vi "SID_1804453_labview_simulation.vi"() -> ()   [LabVIEW 2019]
uses:
  <vilib>/measure/matone.llb/Extract Single Tone Information N Chan.vi
  <vilib>/express/express analysis/Spectral/Block/exnSpectralBlock spectral measurements peak poly.vi
  <vilib>/express/express analysis/Spectral/Block/exnSpectralBlock spectral measurements peak DDT.vi
  <vilib>/express/express analysis/Spectral/XNode/ExpressSpectralMeasurementsBlockNode.xnode
  <vilib>/measure/NI_MAPro.lvlib
panel:
  out "Summing output graph":dynamicdata(graph)
  in  "Frequency":dbl=100.0
  in  "Amplitude":dbl=10.0
  out "peak output":dynamicdata(graph)
  in  "Time Target (s)":dbl=100.0
  out "Elapsed Time (s)":dbl
  in  "Ideal amplitude":dbl
  out "Out of bounds - amplitude":bool
  in  "Ideal frequency":dbl
  out "Out of bounds - frequency":bool
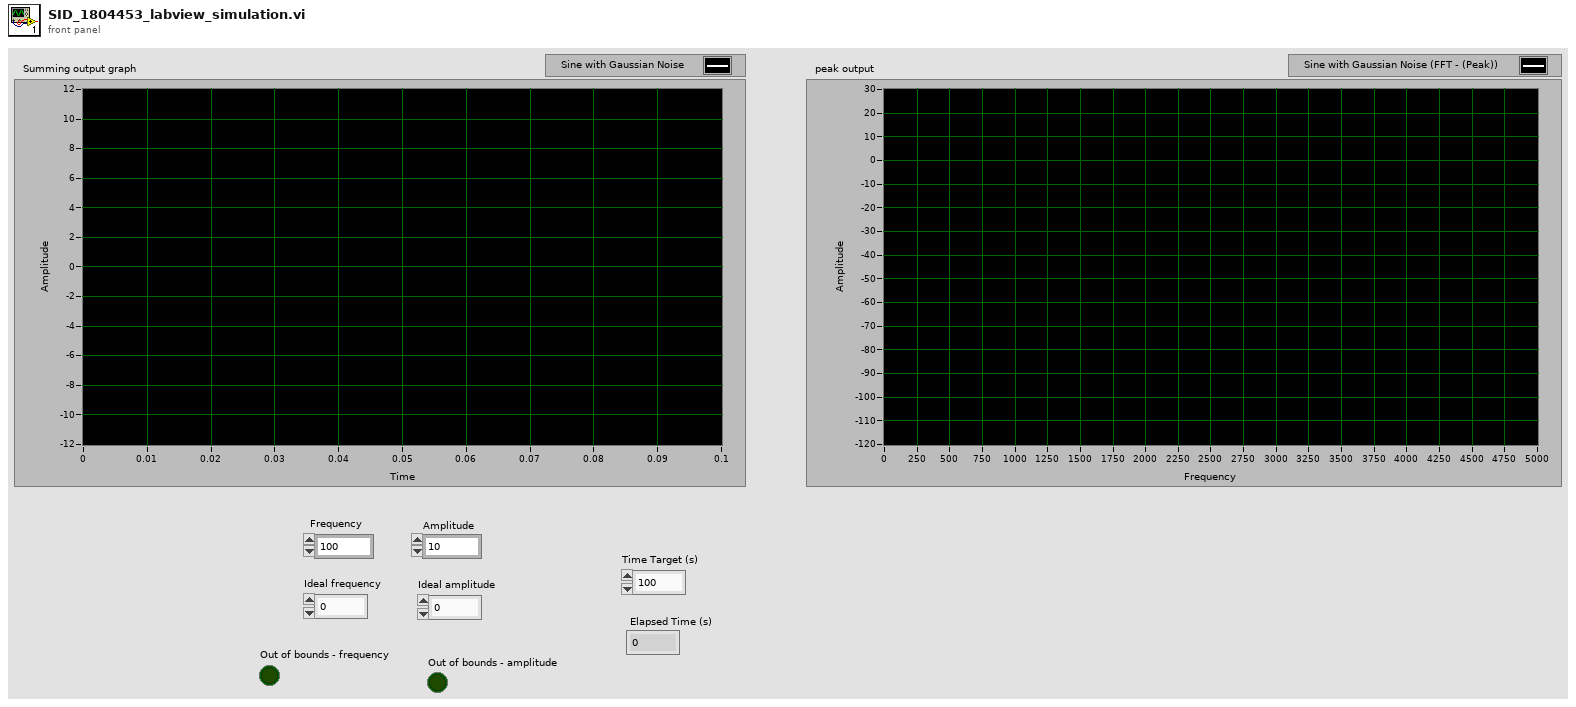
[diagram p1: front panel]
types:
  T1 = cluster{"averaging mode":u16, "weighting mode":u16, "number of averages":u32}
  T2 = cluster{"dB On (F)":bool, "unwrap phase (F)":bool, "convert to degree (F)":bool}
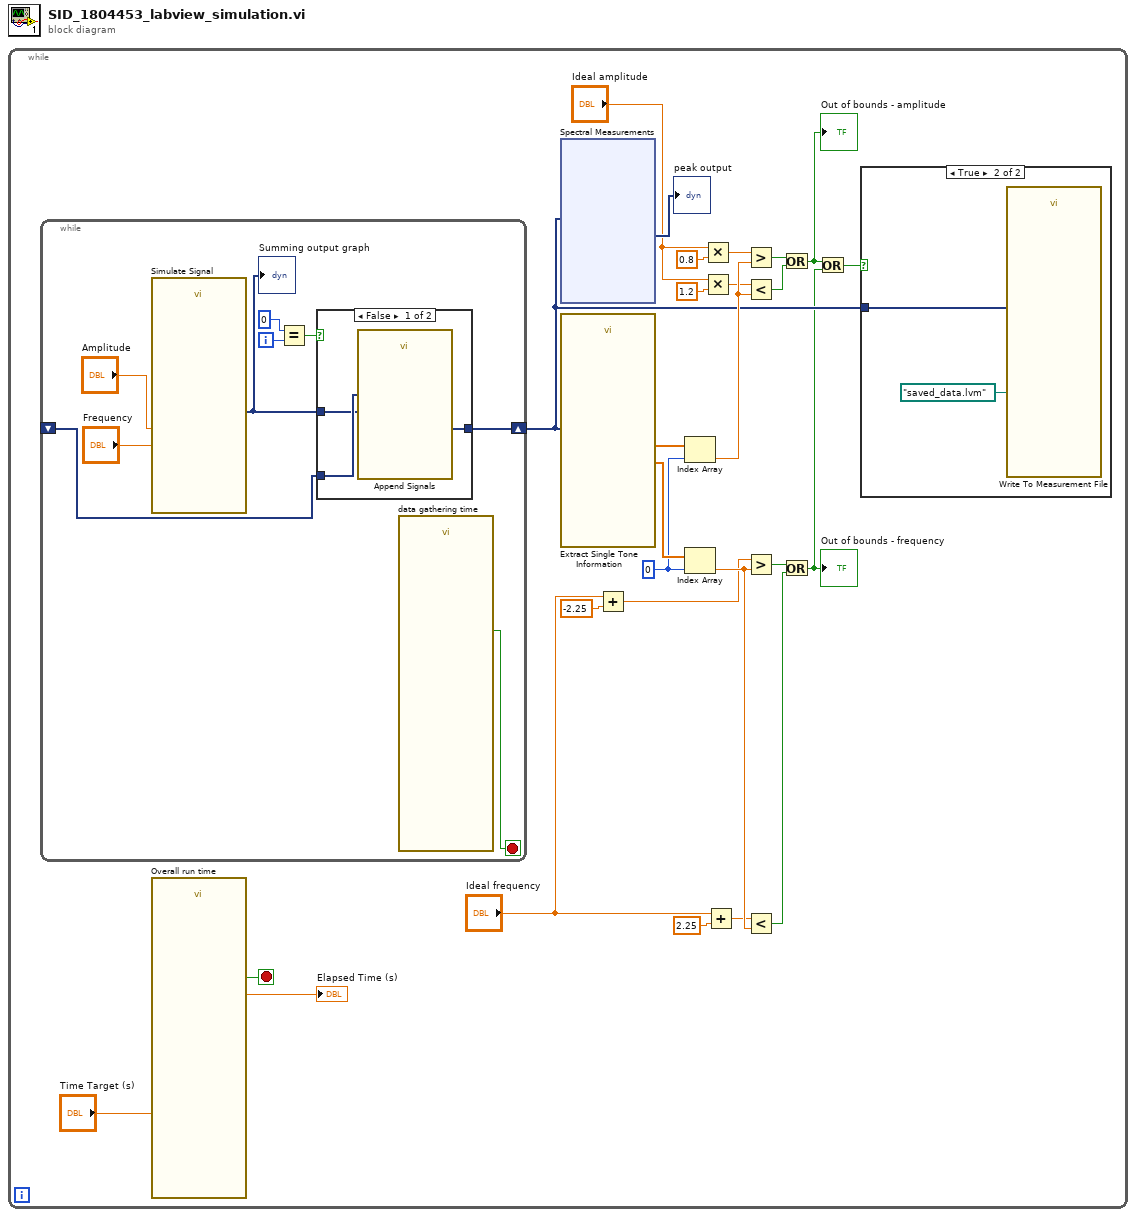
[diagram p0: block diagram]
diagram:
  n1 = while {
    stop <- w26 stop-if-true
    w18 = 0 ("index")
    n2 = while {
      shift-right: [w43] -> w12
      shift-left: _ -> [w44]
      i -> [w46]
      stop <- w48 stop-if-true
      n3 = call "Simulate Signal"("Frequency"="Frequency", "Amplitude"="Amplitude") -> ("Sine with Gaussian Noise"=w40:dynamicdata)  [unwired: 12 in, 1 out]
      "Summing output graph" <- w40
      n4 = Equal?(x=0, y=w46) -> (x = y?=w47:bool)
      n5 = case shown="False" w47 {
        tunnel: [w51 w52] -> w43
        tunnel: w40 -> [w49 w52]
        tunnel: w44 -> [w50 _]
        frame False {
          n6 = call "Append Signals"("Input Signal B"=w49, "Input Signal A"=w50) -> ("Appended Signals"=w51:dynamicdata)  [unwired: 8 in, 1 out]
        }
        frame True {
        }
      }
      n7 = call "data gathering time"() -> ("Time has Elapsed"=w48:bool)  [unwired: 12 in, 7 out]
    }
    n8 = call "Overall run time"("Time Target (s)"="Time Target (s)") -> ("Elapsed Time (s)"=→"Elapsed Time (s)":dbl, "Time has Elapsed"=w26:bool)  [unwired: 11 in, 6 out]
    n9 = xnode "Spectral Measurements"("Signals"=w12) -> ("FFT - (Peak)"=→"peak output":dynamicdata)  [unwired: 1 in, 2 out]
    n10 = call-poly <vilib>:"Extract Single Tone Information.vi"("time signals in"=w12) -> ("detected amplitudes"=w23:dbl[], "detected frequencies"=w22:dbl[])  [unwired: 5 in, 4 out]
    n11 = Add(x="Ideal frequency", y=-2.25) -> (x+y=w4:dbl)
    n12 = Index Array(array=w23, index=w18) -> (element=w15:dbl)
    n13 = Index Array(array=w22, index=w18) -> (element=w9:dbl)
    n14 = Multiply(x="Ideal amplitude", y=0.8) -> (x*y=w14:dbl)
    n15 = Multiply(x="Ideal amplitude", y=1.2) -> (x*y=w13:dbl)
    n16 = Add(x="Ideal frequency", y=2.25) -> (x+y=w3:dbl)
    n17 = Greater?(x=w14, y=w15) -> (0:w17:bool)
    n18 = Less?(x=w13, y=w15) -> (x < y?=w16:bool)
    n19 = Greater?(x=w4, y=w9) -> (0:w11:bool)
    n20 = Less?(x=w3, y=w9) -> (x < y?=w10:bool)
    n21 = Or(x=w17, y=w16) -> (x .or. y?=w1:bool)
    "Out of bounds - amplitude" <- w1
    n22 = Or(x=w11, y=w10) -> (x .or. y?=w2:bool)
    "Out of bounds - frequency" <- w2
    n23 = Or(x=w1, y=w2) -> (x .or. y?=w8:bool)
    n24 = case shown="True" w8 {
      tunnel: w12 -> [_ w29]
      frame False {
      }
      frame True {
        n25 = call "Write To Measurement File"("Signals"=w29, "Filename"=path "saved_data.lvm") -> ()  [unwired: 15 in, 3 out]
      }
    }
  }
